vi "KelvinoxRotator_Open_Queue.vi"(8 "error in (no error)":errorcluster) -> (0 "error out":errorcluster, 2 "queue out":refnum<queue>)   [LabVIEW 2019]
uses:
  Gustav/20T_Dewar_Cluster.ctl
  Global/Global Variables/Queues_global.vi
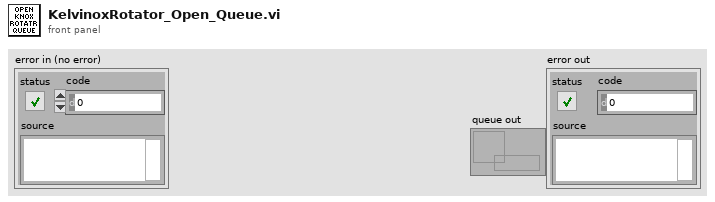
[diagram p1: front panel]
types:
  T1 = typedef "20T_Dewar_Cluster.ctl" = cluster{"Dewar Heater (%) Bar":dbl, "Dewar-Heater (%) Display":dbl, "Dewar-Heater (%) SP":dbl, "Set Dewar-Heater SP":bool, "Change D-Heater Status":bool, "Dewar Pressure":dbl, "Dewar heater manual":bool, "Dewar Heater (W)":dbl}
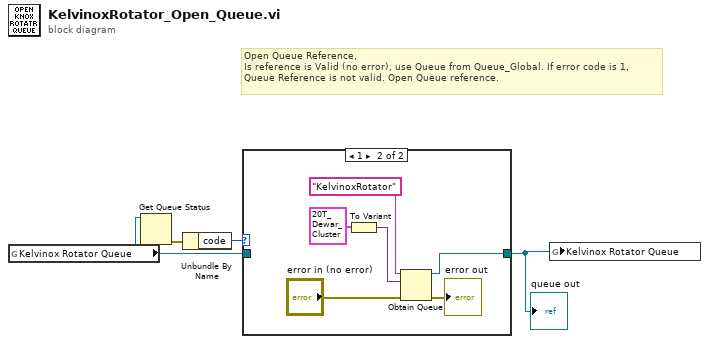
[diagram p0: block diagram]
diagram:
  # "Open Queue Reference, \nIs reference is Valid (no error), use Queue from Queue_Global. If error code is 1, \nQueue Reference is not valid. Open Queue reference."
  n1 = global read "Queues_global.vi" "Kelvinox Rotator Queue"() -> (w2:refnum<queue>)
  n2 = Get Queue Status(queue=w2) -> (error out=w4:errorcluster)  [unwired: 2 in, 7 out]
  n3 = Unbundle By Name(w4) -> ("code"=w3:i32)
  n4 = case shown="1" w3 {
    tunnel: [w5 w7] -> w1
    tunnel: w2 -> [w5 _]
    frame 0, Default {
    }
    frame 1 {
      n5 = To Variant(anything=T1 {"Dewar Heater (%) Bar"=0.0, "Dewar-Heater (%) Display"=3.4572, "Dewar-Heater (%) SP"=0.0, "Set Dewar-Heater SP"=FALSE, "Change D-Heater Status"=FALSE, "Dewar Pressure"=0.0, "Dewar heater manual"=FALSE, "Dewar Heater (W)"=0.0} ("20T-Dewar-Cluster")) -> (Variant=w10:variant)
      n6 = Obtain Queue(name (unnamed)="KelvinoxRotator", element data type=w10, error in (no error)="error in (no error)") -> (queue out=w7:refnum<queue>, error out=→"error out":errorcluster)  [unwired: 2 in, 1 out]
    }
  }
  "queue out" <- w1
  n7 = global write "Queues_global.vi" "Kelvinox Rotator Queue"(w1) -> ()
